vi "Open 6 Motor.vi"(8 "error in (no error)":errorcluster, 11 "Cluster":T1) -> (0 "error out":errorcluster, 3 "RobotDriveDevRef":T2={"DevStatus"={"status"=FALSE, "code"=0, "source"=""}, "Motors[]"=[], "Square Inputs"=FALSE, "Max Output"=1.0})   [LabVIEW 2015]
uses:
  <vilib>/Rock Robotics/WPI/RobotDrive/WPI_RobotDriveDevRef.ctl
  <vilib>/Rock Robotics/WPI/MotorControl/WPI_MotorControlDeviceRef.ctl
  <vilib>/Rock Robotics/WPI/MotorControl/WPI_MotorControlType.ctl
  <vilib>/Rock Robotics/SystemInterfaces/DIO/FPGA_DIOPWMChannel.ctl
  <vilib>/Rock Robotics/WPI/PWM/WPI_PWMDeadband.ctl
  <vilib>/Rock Robotics/WPI/CAN/Jaguar/SubVIs/WPI_CANJaguar_ControlMode.ctl
  <vilib>/Rock Robotics/WPI/CAN/TalonSRX/WPI_CANTalonSRX_APIControlMode.ctl
  <vilib>/Rock Robotics/WPI/SafetyOutput/WPI_SafetyOutputConfigMenu.ctl
  <vilib>/Rock Robotics/WPI/MotorControl/WPI_MotorControlOpenCANTalonSRX.vi
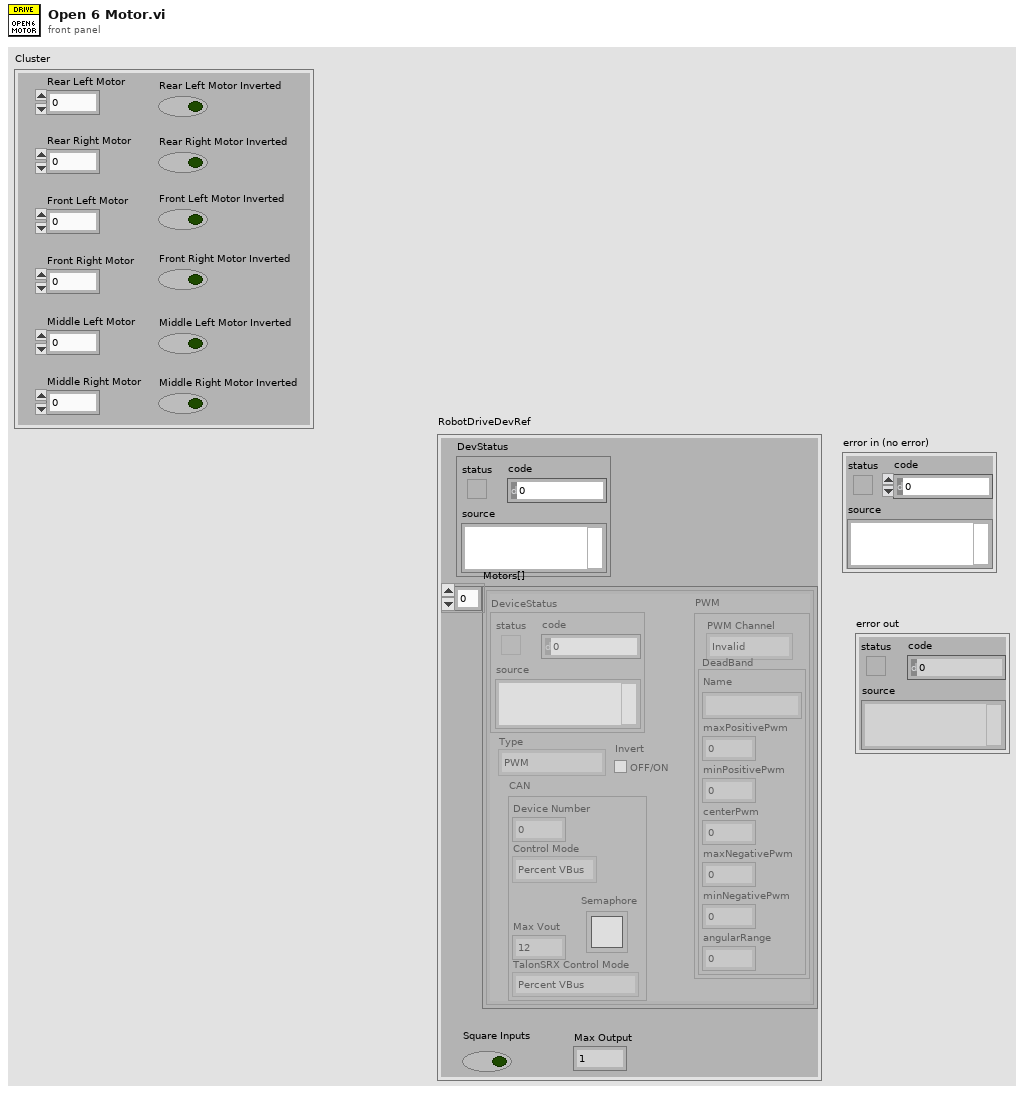
[diagram p1: front panel]
types:
  T1 = cluster{"Front Right Motor Inverted":bool, "Front Left Motor Inverted":bool, "Rear Right Motor Inverted":bool, "Rear Left Motor Inverted":bool, "Middle Right Motor Inverted":bool, "Middle Left Motor Inverted":bool, "Rear Left Motor":u8, "Rear Right Motor":u8, "Front Left Motor":u8, "Front Right Motor":u8, "Middle Left Motor":u8, "Middle Right Motor":u8}
  T2 = typedef "WPI_RobotDriveDevRef.ctl" = cluster{"DevStatus":errorcluster, "Motors[]":T3[], "Square Inputs":bool, "Max Output":dbl}
  T3 = typedef "WPI_MotorControlDeviceRef.ctl" = cluster{"DeviceStatus":errorcluster, "Type":T4, "PWM":cluster{"PWM Channel":T5, "DeadBand":T6}, "CAN":cluster{"Device Number":u8, "Control Mode":T7, "Semaphore":T8, "Max Vout":dbl, "TalonSRX Control Mode":T9}, "Invert":bool}
  T4 = typedef "WPI_MotorControlType.ctl" = enum16{"PWM", "CAN", "CANTalonSRX"}
  T5 = typedef "FPGA_DIOPWMChannel.ctl" = enum8{"PWM 0", "PWM 1", "PWM 2", "PWM 3", "PWM 4", "PWM 5", "PWM 6", "PWM 7", "PWM 8", "PWM 9", "PWM MXP 0", "PWM MXP 1", "PWM MXP 2", "PWM MXP 3", "PWM MXP 4", "PWM MXP 5", "PWM MXP 6", "PWM MXP 7", "PWM MXP 8", "PWM MXP 9", "Invalid"}
  T6 = typedef "WPI_PWMDeadband.ctl" = cluster{"Name":string, "maxPositivePwm":i32, "minPositivePwm":i32, "centerPwm":i32, "maxNegativePwm":i32, "minNegativePwm":i32, "angularRange":u16}
  T7 = typedef "WPI_CANJaguar_ControlMode.ctl" = enum8{"Percent VBus", "Current", "Speed", "Position", "Voltage"}
  T8 = typedef "Semaphore RefNum" = refnum<k1>
  T9 = typedef "WPI_CANTalonSRX_APIControlMode.ctl" = enum8{"Percent VBus", "Speed", "Position", "Slave", "Unchanged / Invalid", "Voltage Compensation", "Current", "Motion Profile"}
  T10 = typedef "WPI_SafetyOutputConfigMenu.ctl" = enum16{"Enable", "Disable"}
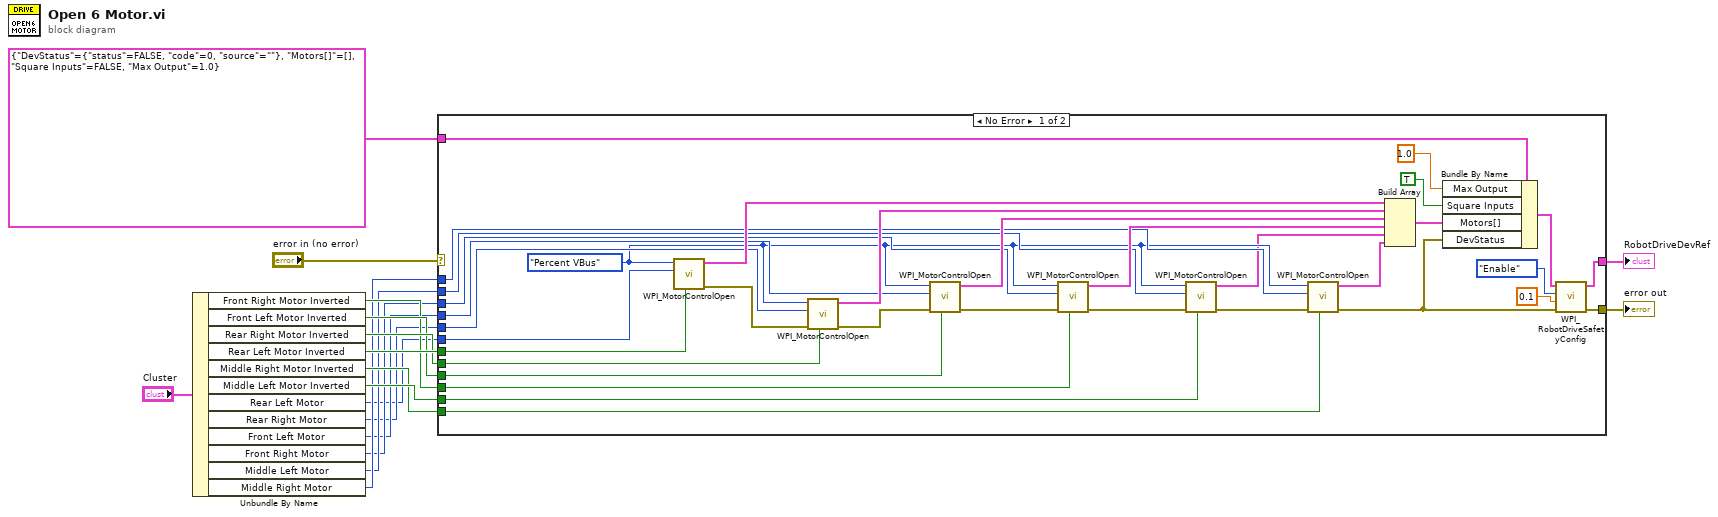
[diagram p0: block diagram]
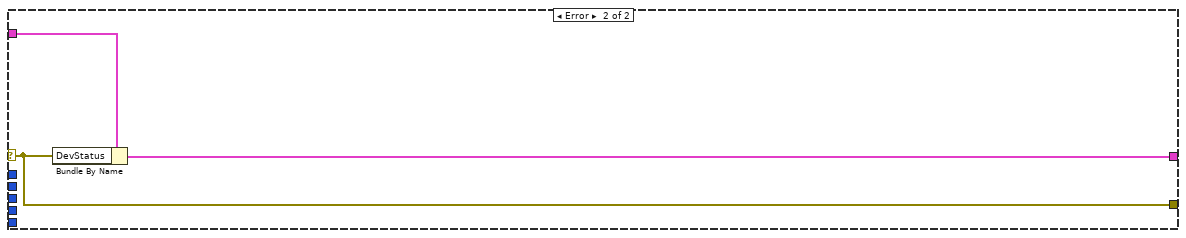
[diagram p2: hidden frame]
diagram:
  n1 = Unbundle By Name("Cluster") -> ("Front Right Motor Inverted"=w9:bool, "Front Left Motor Inverted"=w10:bool, "Rear Right Motor Inverted"=w11:bool, "Rear Left Motor Inverted"=w12:bool, "Middle Right Motor Inverted"=w7:bool, "Middle Left Motor Inverted"=w8:bool, "Rear Left Motor"=w1:u8, "Rear Right Motor"=w2:u8, "Front Left Motor"=w3:u8, "Front Right Motor"=w4:u8, "Middle Left Motor"=w5:u8, "Middle Right Motor"=w6:u8)
  n2 = case shown="No Error" "error in (no error)" {
    selector: "error in (no error)" -> [_ w52]
    tunnel: [w34 w53] -> w14
    tunnel: T2 {"DevStatus"={"status"=FALSE, "code"=0, "source"=""}, "Motors[]"=[], "Square Inputs"=FALSE, "Max Output"=1.0} ("RobotDriveDevRef") -> [w51 w54]
    tunnel: w12 -> [w41 _]
    tunnel: w11 -> [w40 _]
    tunnel: w9 -> [w38 _]
    tunnel: w10 -> [w39 _]
    tunnel: [w35 w52] -> w17
    tunnel: w8 -> [w31 _]
    tunnel: w7 -> [w30 _]
    tunnel: w1 -> [w26 _]
    tunnel: w2 -> [w25 _]
    tunnel: w3 -> [w24 _]
    tunnel: w4 -> [w23 _]
    tunnel: w5 -> [w22 _]
    tunnel: w6 -> [w21 _]
    frame No Error {
      w20 = WPI_CANTalonSRX_APIControlMode."Percent VBus" ("Control Mode")
      n3 = call-poly <vilib>:"WPI_MotorControlOpen.vi"("Invert"=w41, "Device Number"=w26, "Control Mode"=w20) -> ("error out"=w43:errorcluster, "MotorControlDeviceRef"=w49:T3)  [unwired: 2 in, 5 out]
      n4 = call-poly <vilib>:"WPI_MotorControlOpen.vi"("Invert"=w40, "error in (no error)"=w43, "Device Number"=w25, "Control Mode"=w20) -> ("error out"=w44:errorcluster, "MotorControlDeviceRef"=w48:T3)  [unwired: 1 in, 5 out]
      n5 = call-poly <vilib>:"WPI_MotorControlOpen.vi"("Invert"=w39, "error in (no error)"=w44, "Device Number"=w24, "Control Mode"=w20) -> ("error out"=w45:errorcluster, "MotorControlDeviceRef"=w47:T3)  [unwired: 1 in, 5 out]
      n6 = call-poly <vilib>:"WPI_MotorControlOpen.vi"("Invert"=w38, "error in (no error)"=w45, "Device Number"=w23, "Control Mode"=w20) -> ("error out"=w29:errorcluster, "MotorControlDeviceRef"=w46:T3)  [unwired: 1 in, 5 out]
      n7 = call-poly <vilib>:"WPI_MotorControlOpen.vi"("Invert"=w31, "error in (no error)"=w29, "Device Number"=w22, "Control Mode"=w20) -> ("error out"=w28:errorcluster, "MotorControlDeviceRef"=w19:T3)  [unwired: 1 in, 5 out]
      n8 = call-poly <vilib>:"WPI_MotorControlOpen.vi"("Invert"=w30, "error in (no error)"=w28, "Device Number"=w21, "Control Mode"=w20) -> ("error out"=w27:errorcluster, "MotorControlDeviceRef"=w18:T3)  [unwired: 1 in, 5 out]
      n9 = Build Array(w49, w48, w47, w46, w19, w18) -> (w42:T3[])
      n10 = Bundle By Name(cluster=w51, "Max Output"=1.0, "Square Inputs"=TRUE ("DestroyPWM?"), "Motors[]"=w42, "DevStatus"=w27) -> (w36:T2)
      n11 = call <vilib>:"WPI_RobotDriveSafetyConfig.vi"("error in (no error)"=w27, "timeout (s)"=0.1, "mode"=WPI_SafetyOutputConfigMenu."Enable", "RobotDriveDevRef"=w36) -> ("error out"=w35:errorcluster, "RobotDriveDevRef"=w34:T2)  [unwired: 6 out]
    }
    frame Error {
      n12 = Bundle By Name(cluster=w54, "DevStatus"=w52) -> (w53:T2)
    }
  }
  "RobotDriveDevRef" <- w14
  "error out" <- w17
